vi "BS find a tug.vi"(0 "Image Path":T2, 2 "templete path":string="gamma templete.png", 3 "error in":errorcluster, 4 "Greek Letter":string="G") -> (5 "Location":T1, 6 "Valid?":bool, 7 "error out":errorcluster)   [LabVIEW 2012]
doc: "This VI will find the tug with the symbol for the greek letter which is passed. It accepts the pool image and the templete image for the greek letter passed. It outputs the the X and Y location in camera pixels and the heading in degrees. The valid? line indicates the tug was found. If the data is not valid it outputs -1's."
uses:
  <vilib>/vision/Image Controls.llb/IMAQ Image.ctl
panel:
  out "Matches":T3(array[cluster]) {"Bounding Box"."y" format="%.2f"; "Bounding Box"."x" format="%.2f"; "Position"."y" format="%.2f"; "Position"."x" format="%.2f"; "Score" format="%.2f"; "Scale" format="%.2f"; "Angle" format="%.2f"}
  out "Templete Image":T2(plugin-control)
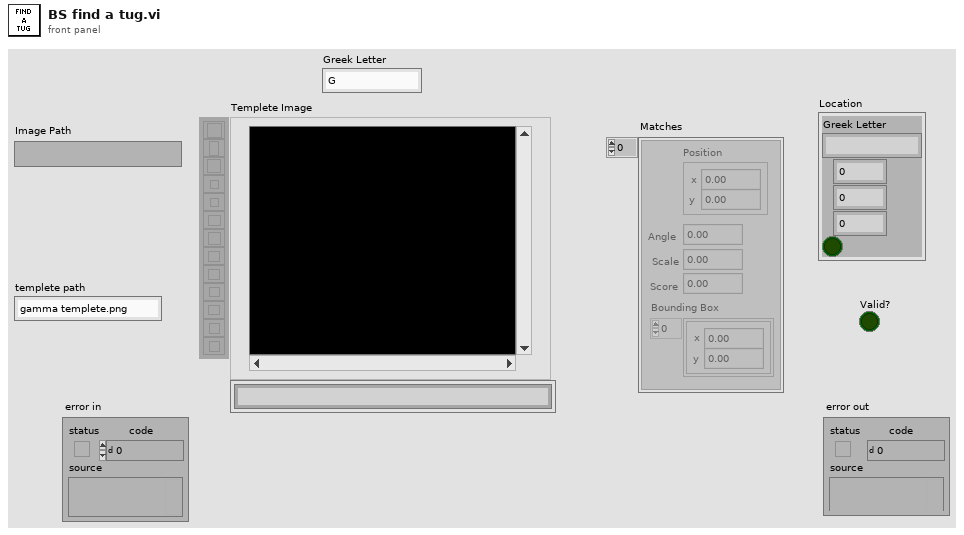
[diagram p1: front panel]
types:
  T1 = cluster{"Greek Letter":string, i16, i16, i16, bool}
  T2 = typedef "IMAQ Image.ctl" = refnum<image>
  T3 = cluster{"Position":cluster{"x":sgl, "y":sgl}, "Angle":sgl, "Scale":sgl, "Score":sgl, "Bounding Box":cluster{"x":sgl, "y":sgl}[]}[]
  T4 = cluster{"Global Rectangle":i32[], "Contours":cluster{"ID":enum32{"External", "Internal"}, "Type":u32, "Coordinates":i32[]}[]}
  T5 = typedef "Image Type" = u32
  T6 = cluster{"Match Mode (Pattern Matching 1)":u16, "Subpixel Accuracy (Pattern Matching 1)":bool, "Rotation Angle Ranges (degrees) (Pattern Matching 1)":cluster{sgl, sgl}[]}
  T7 = cluster{"ROI Descriptor (Pattern Matching 1)":cluster{"Global Rectangle":i32[], "Contours":cluster{"ID":enum32{"External", "Internal"}, "Type":u32, "Coordinates":i32[]}[]}, "Number of Matches Requested (Pattern Matching 1)":i32, "Minimum Match Score (Pattern Matching 1)":sgl}
  T8 = cluster{"Position":cluster{"x":sgl, "y":sgl}, "Angle":sgl, "Scale":sgl, "Score":sgl, "Bounding Box":cluster{"x":sgl, "y":sgl}[]}
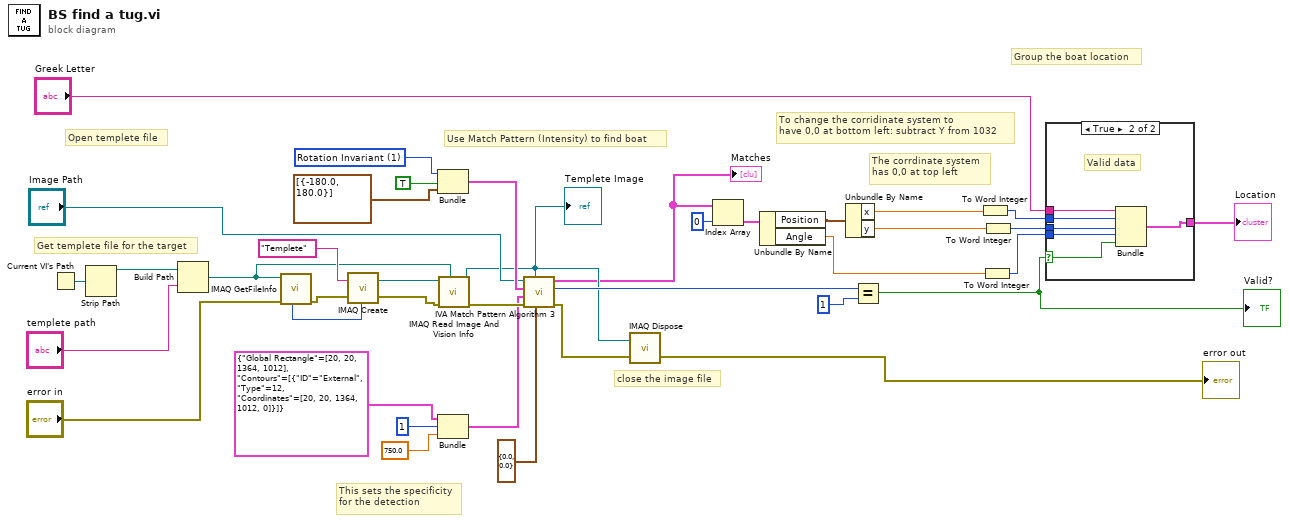
[diagram p0: block diagram]
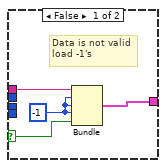
[diagram p2: hidden frame]
diagram:
  w39 = u16 1 items=["Shift Invariant", "Rotation Invariant"] ("Match Mode (Pattern Matching 1)")
  # "This sets the specificity\nfor the detection"
  # "To change the corridinate system to \nhave 0,0 at bottom left: subtract Y from 1032"
  # "The corrdinate system\nhas 0,0 at top left"
  # "Group the boat location"
  # "close the image file"
  # "Use Match Pattern (Intensity) to find boat"
  # "Open templete file"
  # "Get templete file for the target"
  n1 = Current VI's Path() -> (path=w32:path)
  n2 = Strip Path(path=w32) -> (stripped path=w31:path)  [unwired: 1 out]
  n3 = Build Path(base path=w31, name or relative path="templete path") -> (appended path=w27:path)
  n4 = call "IMAQ GetFileInfo"("error in (no error)"="error in", "File Path"=w27) -> ("error out"=w30:errorcluster, "Image Type"=w29:T5)  [unwired: 3 in, 5 out]
  n5 = call "IMAQ Create"("Image Name"="Templete", "Image Type"=w29, "error in (no error)"=w30) -> ("New Image"=w25:T2, "error out"=w26:errorcluster)  [unwired: 1 in, 1 out]
  n6 = Bundle("Match Mode (Pattern Matching 1)"=w39, "Subpixel Accuracy (Pattern Matching 1)"=TRUE, "Rotation Angle Ranges (degrees) (Pattern Matching 1)"=cluster{sgl, sgl}[] [{-180.0, 180.0}]) -> (w22:T6)  [unwired: 1 out]
  n7 = Bundle("ROI Descriptor (Pattern Matching 1)"=T4 {"Global Rectangle"=[20, 20, 1364, 1012], "Contours"=[{"ID"=enum."External", "Type"=12, "Coordinates"=[20, 20, 1364, 1012, 0]}]}, "Number of Matches Requested (Pattern Matching 1)"=1, "Minimum Match Score (Pattern Matching 1)"=sgl 750.0) -> (w23:T7)  [unwired: 1 out]
  n8 = call "IMAQ Read Image And Vision Info"("File Path"=w27, "error in (no error)"=w26, "Image"=w25) -> ("error out"=w24:errorcluster, "Image Out"=w3:T2)  [unwired: 1 in, 6 out]
  "Templete Image" <- w3
  n9 = call <vilib>:"IVA Match Pattern Algorithm 3.vi"("Match Offset"=cluster{"X":sgl, "Y":sgl} {"X"=0.0, "Y"=0.0} ("Match Offset (Pattern Matching 1)"), "Image Template"=w3, "error in (no error)"=w24, "Match Parameters"=w23, "Setup Match Parameters"=w22, "Image"="Image Path") -> ("error out"=w8:errorcluster, "Number of Matches"=w12:i32, "Matches"=w2:T3)  [unwired: 3 out]
  "Matches" <- w2
  n10 = call "IMAQ Dispose"("Image"=w3, "error in (no error)"=w8) -> ("error out"=→"error out":errorcluster)  [unwired: 4 in]
  n11 = Index Array(array=w2, index=0) -> (element=w20:T8)
  n12 = Unbundle By Name(w20) -> ("Position"=w19:cluster{"x":sgl, "y":sgl}, "Angle"=w16:sgl)
  n13 = Unbundle By Name(w19) -> ("x"=w17:sgl, "y"=w1:sgl)
  n14 = Equal?(x=w12, y=1) -> (x = y?=w6:bool)
  "Valid?" <- w6
  n15 = To Word Integer(number=w17) -> (16bit integer=w15:i16)
  n16 = To Word Integer(number=w16) -> (16bit integer=w13:i16)
  n17 = To Word Integer(number=w1) -> (16bit integer=w14:i16)
  n18 = case shown="True" w6 {
    selector: w6 -> [w40 w45]
    tunnel: "Greek Letter" -> [w43 w49]
    tunnel: w15 -> [_ w48]
    tunnel: w14 -> [_ w47]
    tunnel: w13 -> [_ w46]
    tunnel: [w41 w44] -> w4
    frame False {
      w42 = i16 -1
      # "Data is not valid\nload -1's"
      n19 = Bundle("Greek Letter"=w43, w42, w42, w42, w40) -> (w41:T1)  [unwired: 1 in]
    }
    frame True {
      # "Valid data"
      n20 = Bundle("Greek Letter"=w49, w48, w47, w46, w45) -> (w44:T1)  [unwired: 1 in]
    }
  }
  "Location" <- w4
